vi "Relay - Message Mode.vi"(8 "error in (no error)":errorcluster) -> (0 "error out":errorcluster)   [LabVIEW 2026, in "Tests.lvlib"]
doc: "Verifies RelayAppender message mode forwards each accepted statement as a LogStatementMsg to the application-supplied consumer enqueuer (SRS-LMBR-024). A queue-mode relay is launched standalone as the consumer; a message-mode relay is registered with the manager pointing at the consumer's enqueuer. One Info statement is logged, and the test asserts it arrives intact in the consumer's queue exactly once. Integration tier; runs sequentially.\n\nImplements LMBR-T-043 -> SRS-024. Assert-level IDs: Test-ID-Assert-Checklist.md."
uses:
  Tests.lvlib
  src/TypeDefs/Severity.ctl
  src/TypeDefs/AppenderConfig.ctl
  src/TypeDefs/Filter.ctl
  src/TypeDefs/FilterMode.ctl
  src/TypeDefs/DropPolicy.ctl
  src/TypeDefs/RelayMode.ctl
  src/Core/Appenders/RelayAppender.lvclass/RelayAppender.lvclass
  <vilib>/ActorFramework/Message Enqueuer/Message Enqueuer.lvclass/Message Enqueuer.ctl
  <vilib>/ActorFramework/Message Enqueuer/Enqueue.vi
  <vilib>/ActorFramework/Stop Msg/Stop Msg.lvclass
  <vilib>/addons/_JKI Toolkits/Caraya/classes/Assert/Assert False.vi
  <vilib>/addons/_JKI Toolkits/Caraya/classes/Assert/Assert Equal Value_Variant.vi
  <vilib>/addons/_JKI Toolkits/Caraya/classes/Assert/Assert True.vi
  <vilib>/ActorFramework/Message Priority Queue/Priority Enqueue.vi
  <vilib>/addons/_JKI Toolkits/Caraya/classes/Test/Test.lvclass
  src/Lumberjack.lvlib
  src/Public/Logger.lvclass/Logger.lvclass
  <vilib>/addons/_JKI Toolkits/Caraya/classes/Assert/Assert.lvclass
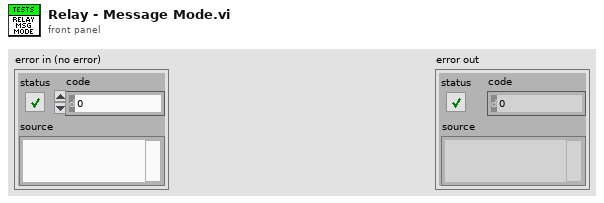
[diagram p1: front panel]
types:
  T1 = typedef "Lumberjack.lvlib/Severity.ctl" = enum16{"OFF", "FATAL", "ERROR", "WARN", "INFO", "DEBUG", "TRACE", "ALL"}
  T2 = typedef "Lumberjack.lvlib/RelayMode.ctl" = enum16{"Message", "Queue"}
  T3 = typedef "Lumberjack.lvlib/AppenderConfig.ctl" = cluster{"id":string, "threshold":T1, "filter":T4, "queueBound":i32, "dropPolicy":T6, "useUTC":bool}
  T4 = typedef "Lumberjack.lvlib/Filter.ctl" = cluster{"mode":T5, "levelMin":T1, "levelMax":T1, "tagPrefix":string}
  T5 = typedef "Lumberjack.lvlib/FilterMode.ctl" = enum16{"Mirror", "Routed"}
  T6 = typedef "Lumberjack.lvlib/DropPolicy.ctl" = enum16{"DropOldest", "DropNewest", "LevelAware"}
  T7 = typedef "Lumberjack.lvlib/Statement.ctl" = cluster{"timestamp":timestamp, "level":T1, "sourceTag":string, "originVI":string, "message":string}
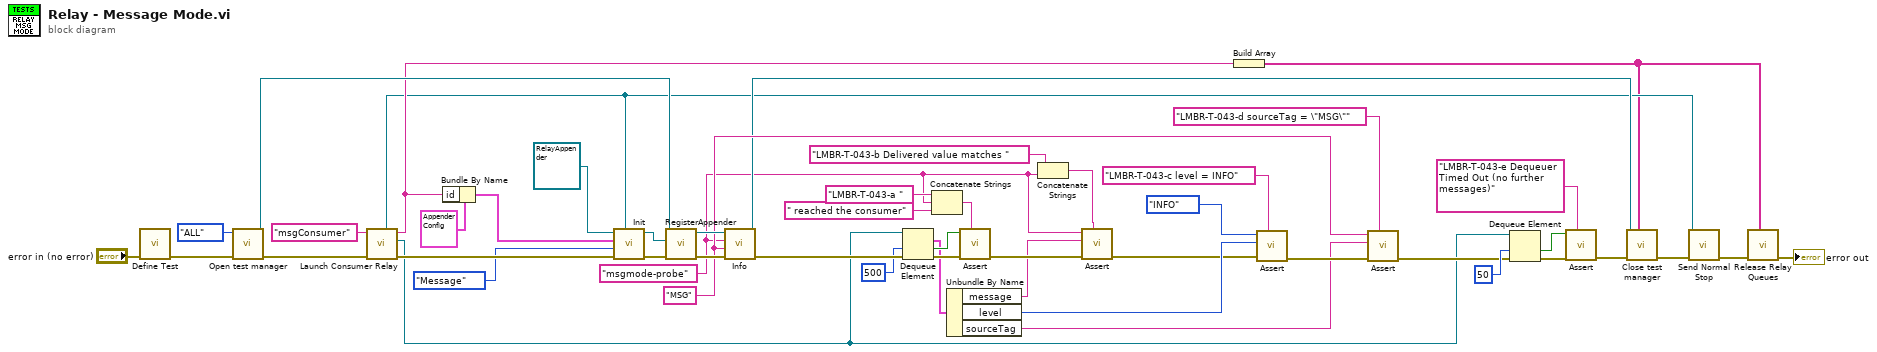
[diagram p0: block diagram]
diagram:
  w21 = "MSG" ("sourceTag")
  w2 = "msgmode-probe" ("message")
  n1 = call <vilib>:"Define Test.vi"("error in (no error)"="error in (no error)") -> ("error out"=w49:errorcluster)  [unwired: 9 in, 1 out]
  n2 = call "Open test manager.vi"("error in (no error)"=w49, "globalThreshold"=Severity."ALL") -> ("error out"=w47:errorcluster, "Logger out"=w13:refnum<class "Logger.lvclass">)  [unwired: 8 in]
  n3 = call "Launch Consumer Relay.vi"("error in (no error)"=w47, "id in"="msgConsumer") -> ("error out"=w44:errorcluster, "consumerQueue"=w18:refnum<queue>, "id out"=w11:string, "consumerEnqueuer"=w9:refnum<class "Message Enqueuer.lvclass">)  [unwired: 6 in]
  n4 = Bundle By Name(cluster=T3 {"id"="", "threshold"=enum."INFO", "filter"={"mode"=enum."Mirror", "levelMin"=enum."INFO", "levelMax"=enum."INFO", "tagPrefix"=""}, "queueBound"=0, "dropPolicy"=enum."DropOldest", "useUTC"=FALSE} ("AppenderConfig"), "id"=w11) -> (w42:T3)
  n5 = call "Init.vi"("Enqueuer in"=w9, "error in (no error)"=w44, "mode"=RelayMode."Message", "common"=w42, "RelayAppender in"=refnum<class "RelayAppender.lvclass"> refnum) -> ("error out"=w43:errorcluster, "RelayAppender out"=w41:refnum<class "RelayAppender.lvclass">)  [unwired: 5 in]
  n6 = call "RegisterAppender.vi"("error in (no error)"=w43, "Lumberjack.lvlib:Appender.lvclass"=w41, "Logger in"=w13) -> ("error out"=w40:errorcluster, "Logger out"=w39:refnum<class "Logger.lvclass">)  [unwired: 7 in]
  n7 = call "Info.vi"("error in (no error)"=w40, "sourceTag"=w21, "message"=w2, "Logger in"=w39) -> ("error out"=w37:errorcluster, "Logger out"=w12:refnum<class "Logger.lvclass">)  [unwired: 6 in]
  n8 = Dequeue Element(queue=w18, timeout in ms (-1)=500, error in (no error)=w37) -> (element=w30:T7, timed out?=w35:bool, error out=w34:errorcluster)  [unwired: 1 out]
  n9 = Concatenate Strings("LMBR-T-043-a " ("Label"), w2, " reached the consumer" ("Label")) -> (w32:string)
  n10 = Unbundle By Name(w30) -> ("message"=w25:string, "level"=w29:T1, "sourceTag"=w22:string)
  n11 = call-poly <vilib>:"Assert.vi"("Label"=w32, "error in (no error)"=w34, "False?"=w35) -> ("error out"=w31:errorcluster)  [unwired: 7 in, 1 out]
  n12 = Concatenate Strings("LMBR-T-043-b Delivered value matches " ("Label"), w2) -> (w1:string)
  n13 = call-poly <vilib>:"Assert.vi"("Label"=w1, "error in (no error)"=w31, "Actual"=w25, "Expected"=w2) -> ("error out"=w26:errorcluster)  [unwired: 6 in, 1 out]
  n14 = Build Array(w11) -> (w7:string[])
  n15 = call-poly <vilib>:"Assert.vi"("Label"="LMBR-T-043-c level = INFO", "error in (no error)"=w26, "Actual"=w29, "Expected"=Severity."INFO" ("globalThreshold")) -> ("error out"=w23:errorcluster)  [unwired: 6 in, 1 out]
  n16 = call-poly <vilib>:"Assert.vi"("Label"="LMBR-T-043-d sourceTag = \"MSG\"", "error in (no error)"=w23, "Actual"=w22, "Expected"=w21) -> ("error out"=w19:errorcluster)  [unwired: 6 in, 1 out]
  n17 = Dequeue Element(queue=w18, timeout in ms (-1)=50, error in (no error)=w19) -> (timed out?=w16:bool, error out=w17:errorcluster)  [unwired: 2 out]
  n18 = call-poly <vilib>:"Assert.vi"("Label"="LMBR-T-043-e Dequeuer Timed Out (no further messages)", "error in (no error)"=w17, "True?"=w16) -> ("error out"=w14:errorcluster)  [unwired: 7 in, 1 out]
  n19 = call "Close test manager.vi"("queueIDList"=w7, "error in (no error)"=w14, "Logger in"=w12) -> ("error out"=w10:errorcluster)  [unwired: 6 in]
  n20 = call <vilib>:"Send Normal Stop.vi"("error in (no error)"=w10, "Message Enqueuer"=w9) -> ("error out"=w8:errorcluster)  [unwired: 9 in]
  n21 = call "Release Relay Queues.vi"("queueIDList"=w7, "error in (no error)"=w8) -> ("error out"=→"error out":errorcluster)  [unwired: 7 in]
